vi "KISSIA_PARSE_MIDE_CELDAS.vi"(11 "String":string="Mide Celda GAS 1, mide Celda H2S 1,  y pausa 0.2s") -> (1 "Pausa (s)":dbl=1.0, 2 "Mide Celda H2S":bool=TRUE, 3 "Mide Celda GAS":bool=TRUE)   [LabVIEW 2017]
panel:
  # "Mide Celda GAS 1, mide Celda H2S 1,  y pausa 0.2s"
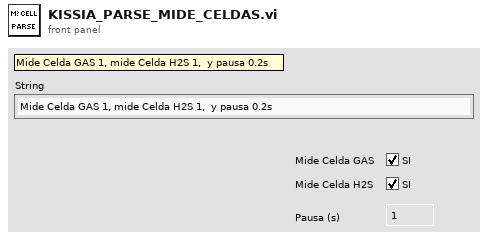
[diagram p1: front panel]
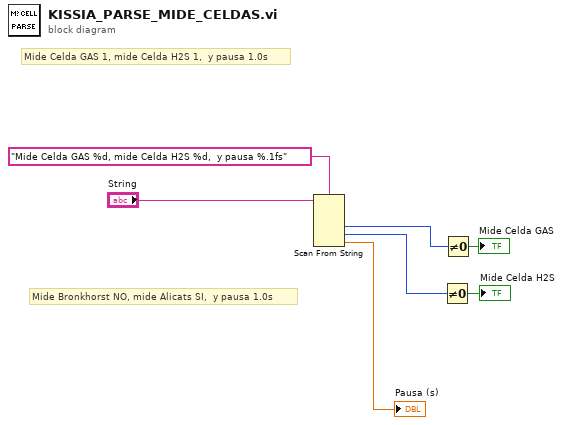
[diagram p0: block diagram]
diagram:
  # "Mide Celda GAS 1, mide Celda H2S 1,  y pausa 1.0s"
  # "Mide Bronkhorst NO, mide Alicats SI,  y pausa 1.0s"
  n1 = Scan From String(format string="Mide Celda GAS %d, mide Celda H2S %d,  y pausa %.1fs", input string="String") -> (output 1=w4:i32, output 2=w1:i32, output 3=→"Pausa (s)":dbl)  [unwired: 5 in, 3 out]
  n2 = Not Equal To 0?(x=w1) -> (x != 0?=→"Mide Celda H2S":bool)
  n3 = Not Equal To 0?(x=w4) -> (x != 0?=→"Mide Celda GAS":bool)
